vi "HF turbidimeter (com4).vi"(4 "State":i16, 5 "Time":dbl format="%.2f", 6 "Sensor Values":dbl[](array[numeric]), 7 "Set Points":dbl[](array[numeric])) -> (0 "required data":T2={"Set Point names"=["unitID (usually 1)"], "required number of setpoints"=1, "required number of sensors"=0, "Sensor names"=[]}, 3 "output value":dbl)   [LabVIEW 2019]
panel:
  in  "error in (no error)":errorcluster
  out "Previous data":T1(array[cluster])
  out "all bad":bool
  out "x-1":i32
  out "UnitID":i32
  out "write buffer":string
  out "Numeric":i32
  # "Enter the correct information for this control code in the required data structure below. Then make the current value default by right clicking on the border of the data structure. Select \"data operations\" and then select \"make current value default\". These values will be displayed by process controller."
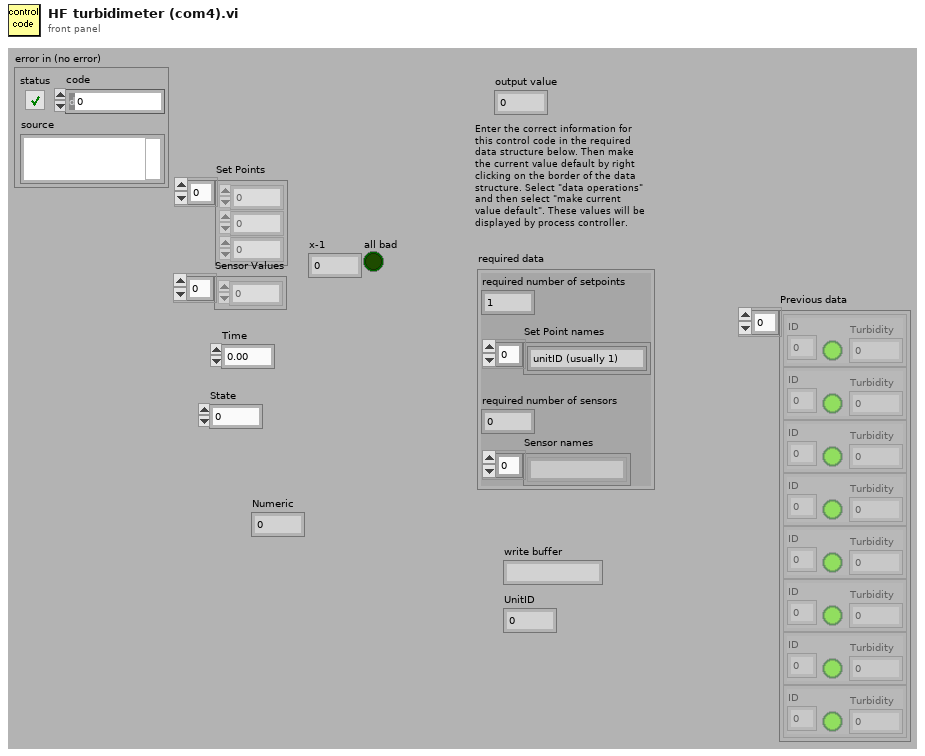
[diagram p1: front panel]
types:
  T1 = cluster{"ID":dbl, "Failed":bool, "Turbidity":dbl}[]
  T2 = cluster{"Set Point names":string[], "required number of setpoints":u8, "required number of sensors":u8, "Sensor names":string[]}
  T3 = cluster{"ID":dbl, "Failed":bool, "Turbidity":dbl}
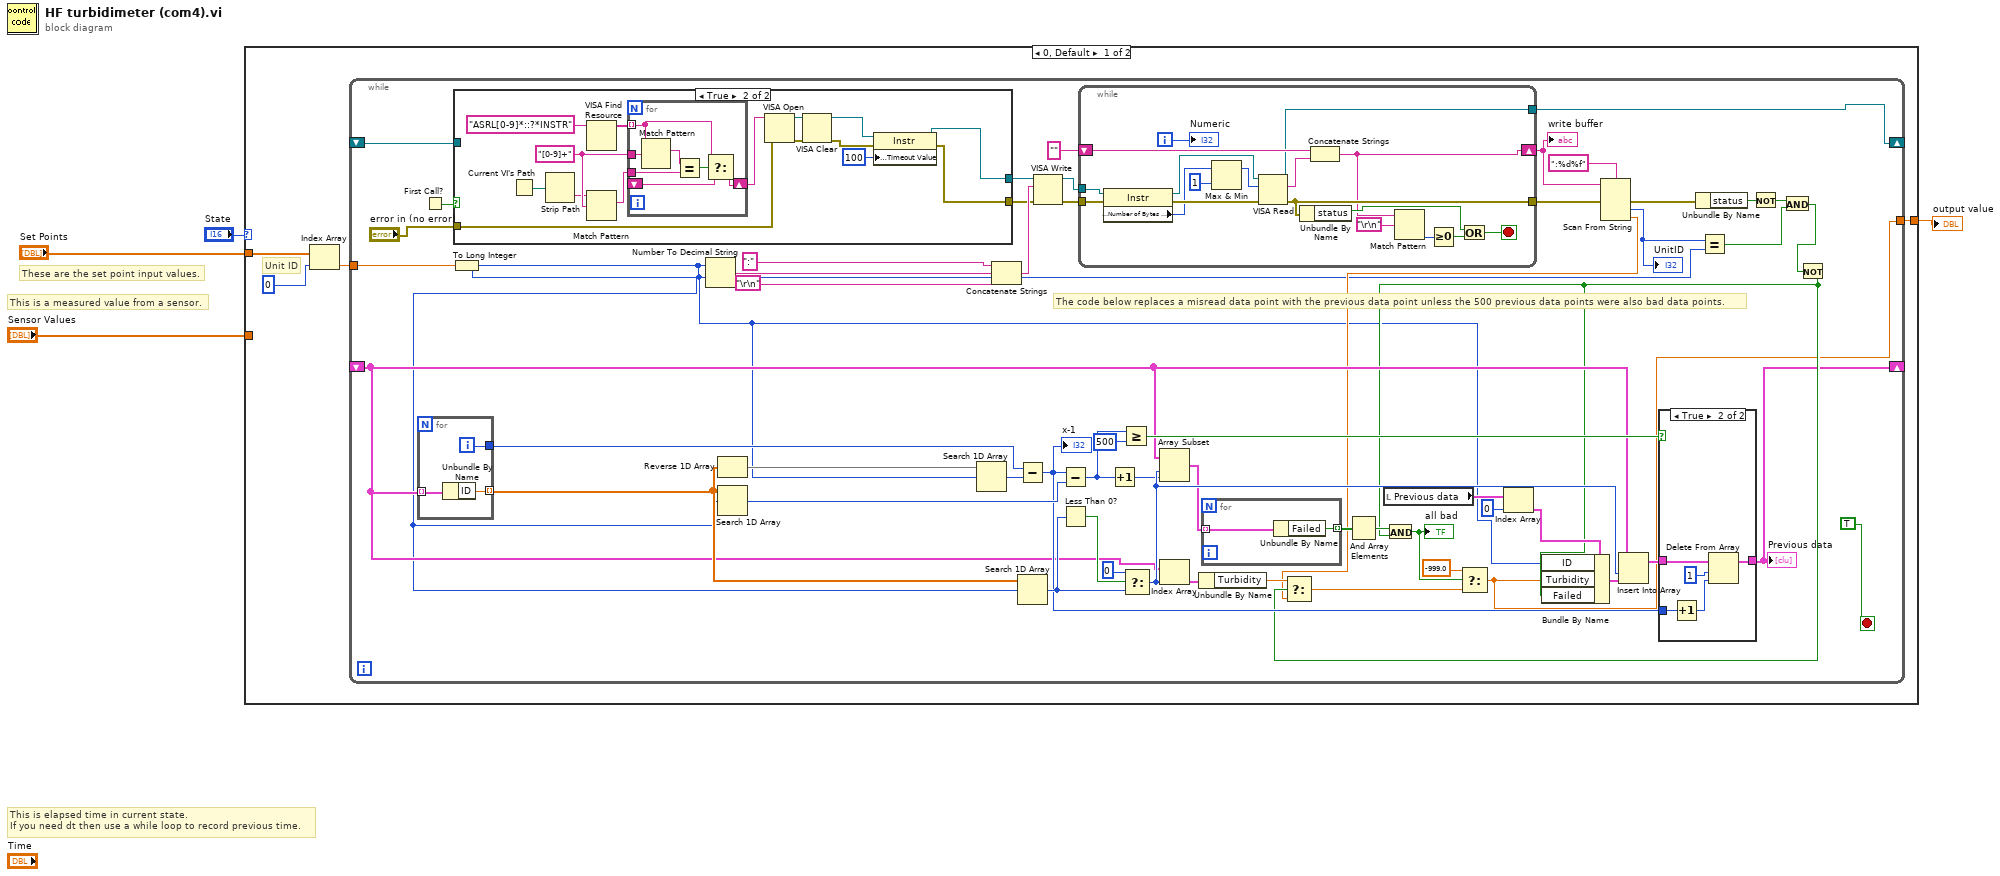
[diagram p0: block diagram]
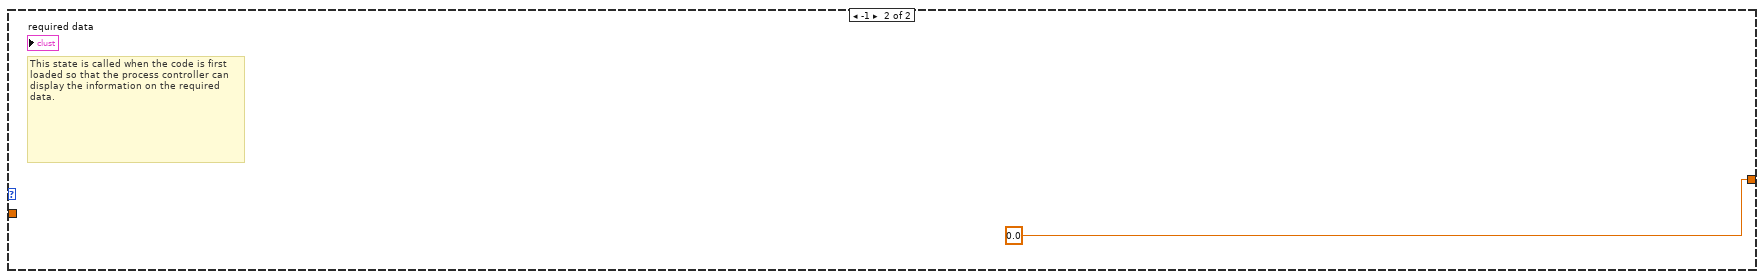
[diagram p4: hidden frame]
diagram:
  # "These are the set point input values."
  # "This is a measured value from a sensor."
  # "This is elapsed time in current state.\nIf you need dt then use a while loop to record previous time."
  n1 = case shown="0, Default" "State" {
    tunnel: [w5 0.0 ("fraction on")] -> w3
    tunnel: "Set Points" -> [w7 _]
    tunnel: "Sensor Values" -> [_ _]
    frame 0, Default {
      # "Unit ID"
      n2 = Index Array(array=w7, index=0) -> (element=w6:dbl)
      n3 = while {
        tunnel: w6 -> [w54]
        tunnel: [w14] -> w5
        shift-right: [w13] -> _
        shift-left: _ -> [w19]
        shift-right: [w10] -> _
        shift-left: _ -> [w9]
        stop <- TRUE stop-if-true
        # "The code below replaces a misread data point with the previous data point unless the 500 previous data points were also bad data points."
        n4 = for {
          tunnel: w19 -> [w70] mode=indexing
          tunnel: [w69] -> w26 mode=indexing
          tunnel: [w68] -> w25
          i -> [w68]
          n5 = Unbundle By Name(w70) -> ("ID"=w69:dbl)
        }
        n6 = First Call?() -> (First Call?: T/F=w56:bool)
        n7 = To Long Integer(number=w54) -> (32bit integer=w15:i32)
        n8 = case shown="True" w56 {
          tunnel: [w77 w82] -> w64
          tunnel: [w78 w81] -> w12
          tunnel: "error in (no error)" -> [w78 w84]
          tunnel: w9 -> [w77 _]
          frame False {
          }
          frame True {
            w93 = "[0-9]+" ("regular expression")
            n9 = Current VI's Path() -> (path=w88:path)
            n10 = Strip Path(path=w88) -> (name=w89:string)  [unwired: 1 out]
            n11 = VISA Find Resource(11:"ASRL[0-9]*::?*INSTR" ("expression (\"?*\")")) -> (3:w91:string[])  [unwired: 2 in, 2 out]
            n12 = Match Pattern(string=w89, regular expression=w93) -> (match substring=w92:string)  [unwired: 1 in, 3 out]
            n13 = for {
              tunnel: w91 -> [w95] mode=indexing
              tunnel: w92 -> [w99]
              shift-right: [w96] -> w87
              shift-left: _ -> [w97]
              tunnel: w93 -> [w94]
              n14 = Match Pattern(string=w95, regular expression=w94) -> (match substring=w100:string)  [unwired: 1 in, 3 out]
              n15 = Equal?(x=w100, y=w99) -> (x = y?=w98:bool)
              n16 = Select(t=w95, s=w98, f=w97) -> (s? t:f=w96:string)
            }
            n17 = VISA Open(error in (no error)=w84, VISA resource name=w87) -> (VISA resource name=w86:refnum<visa-resource-name>, error out=w85:errorcluster)  [unwired: 3 in]
            n18 = VISA Clear(VISA resource name=w86, error in (no error)=w85) -> (VISA resource name out=w83:refnum<visa-resource-name>, error out=w80:errorcluster)
            n19 = property class="Instr"(reference=w83, error in=w80, "General Settings:Timeout Value"=u32 100) -> (reference out=w82:refnum<visa-resource-name>, error out=w81:errorcluster)
          }
        }
        n20 = Number To Decimal String(number=w15) -> (decimal integer string=w57:string)  [unwired: 1 in]
        n21 = Reverse 1D Array(array=w26) -> (reversed array=w42:dbl[])
        n22 = Search 1D Array(1D array=w26, element=w15) -> (index of element=w38:i32)  [unwired: 1 in]
        n23 = Search 1D Array(1D array=w42, element=w15) -> (index of element=w41:i32)  [unwired: 1 in]
        n24 = Concatenate Strings(":" ("string"), w57, "\r\n") -> (w60:string)
        n25 = Subtract(x=w25, y=w41) -> (x-y=w32:i32)
        "x-1" <- w32
        n26 = Search 1D Array(1D array=w26, element=w15) -> (index of element=w36:i32)  [unwired: 1 in]
        n27 = VISA Write(VISA resource name=w64, write buffer=w60, error in (no error)=w12) -> (VISA resource name out=w63:refnum<visa-resource-name>, error out=w62:errorcluster)  [unwired: 1 out]
        n28 = Subtract(x=w32, y=w38) -> (x-y=w29:i32)
        n29 = Less Than 0?(x=w36) -> (x < 0?=w37:bool)
        n30 = while {
          tunnel: w63 -> [w117]
          tunnel: w62 -> [w115]
          shift-right: [w102] -> w50
          shift-left: "" ("write buffer") -> [w118]
          tunnel: [w104] -> w53
          tunnel: [w101] -> w10
          i -> [w103]
          stop <- w113 stop-if-true
          n31 = property class="Instr"(reference=w117, error in=w115) -> (reference out=w116:refnum<visa-resource-name>, error out=w114:errorcluster, "Serial Settings:Number of Bytes at Serial Port"=w106:u32)
          n32 = Max & Min(x=w106, y=u32 1) -> (max(x,y)=w107:u32)  [unwired: 1 out]
          n33 = VISA Read(VISA resource name=w116, byte count=w107, error in (no error)=w114) -> (VISA resource name out=w101:refnum<visa-resource-name>, read buffer=w111:string, error out=w104:errorcluster)  [unwired: 1 out]
          n34 = Unbundle By Name(w104) -> ("status"=w112:bool)
          n35 = Concatenate Strings(w118, w111) -> (w102:string)
          n36 = Match Pattern(string=w102, regular expression="\r\n") -> (offset past match=w109:i32)  [unwired: 1 in, 3 out]
          n37 = Greater Or Equal To 0?(x=w109) -> (x >= 0?=w108:bool)
          n38 = Or(x=w112, y=w108) -> (x .or. y?=w113:bool)
          "Numeric" <- w103
        }
        "write buffer" <- w50
        n39 = Increment(x=w29) -> (x+1=w28:i32)
        n40 = Greater Or Equal?(x=w29, y=500) -> (x >= y?=w39:bool)
        n41 = Select(t=0 ("index of element"), s=w37, f=w36) -> (s? t:f=w30:i32)
        n42 = Array Subset(array=w19, index=w30, length=w28) -> (w27:T1)
        n43 = Index Array(array=w19, index=w30) -> (element=w34:T3)
        n44 = Unbundle By Name(w34) -> ("Turbidity"=w33:dbl)
        n45 = for {
          tunnel: w27 -> [w67] mode=indexing
          tunnel: [w66] -> w24 mode=indexing
          n46 = Unbundle By Name(w67) -> ("Failed"=w66:bool)
        }
        n47 = And Array Elements(Boolean array=w24) -> (logical AND=w21:bool)
        n48 = local read "Previous data"() -> (w46:T1)
        n49 = Index Array(array=w46, index=0) -> (element=w44:T3)
        n50 = Scan From String(format string=":%d%f", input string=w50, error in=w53) -> (error out=w52:errorcluster, output 1=w49:i32, output 2=w16:dbl)  [unwired: 3 in, 2 out]
        "UnitID" <- w49
        n51 = Unbundle By Name(w52) -> ("status"=w51:bool)
        n52 = Equal?(x=w49, y=w15) -> (x = y?=w47:bool)
        n53 = Not(x=w51) -> (.not. x?=w48:bool)
        n54 = And(x=w48, y=w47) -> (x .and. y?=w18:bool)
        n55 = Not(x=w18) -> (.not. x?=w17:bool)
        n56 = Select(t=w33, s=w17, f=w16) -> (s? t:f=w22:dbl)
        n57 = And(x=w21, y=w17) -> (x .and. y?=w20:bool)
        "all bad" <- w20
        n58 = Select(t=-999.0, s=w20, f=w22) -> (s? t:f=w14:dbl)
        n59 = Bundle By Name(cluster=w44, "ID"=w15, "Turbidity"=w14, "Failed"=w17) -> (w43:T3)
        n60 = Insert Into Array(array=w19, index=w30, new element=w43) -> (w31:T1)
        n61 = case shown="True" w39 {
          tunnel: w31 -> [w71 w76]
          tunnel: [w71 w75] -> w13
          tunnel: w32 -> [_ w74]
          frame False {
          }
          frame True {
            n62 = Increment(x=w74) -> (x+1=w72:i32)
            n63 = Delete From Array(array=w76, length=1, index=w72) -> (array with subset deleted=w75:T1)  [unwired: 1 out]
          }
        }
        "Previous data" <- w13
      }
    }
    frame -1 {
      # "This state is called when the code is first loaded so that the process controller can display the information on the required data."
    }
  }
  "output value" <- w3
